vi "adc_plot.vi"(0 "Ch0":dbl[](array[numeric]), 1 "CH1":dbl[](array[numeric]), 2 "CH2":dbl[](array[numeric]), 3 "CH3":dbl[](array[numeric]), 4 "time":dbl[](array[numeric])) -> (7 "XY Graph":cluster{"time 2":dbl[], "Ch0":dbl[]}[](graph))   [LabVIEW 2022 SP3]
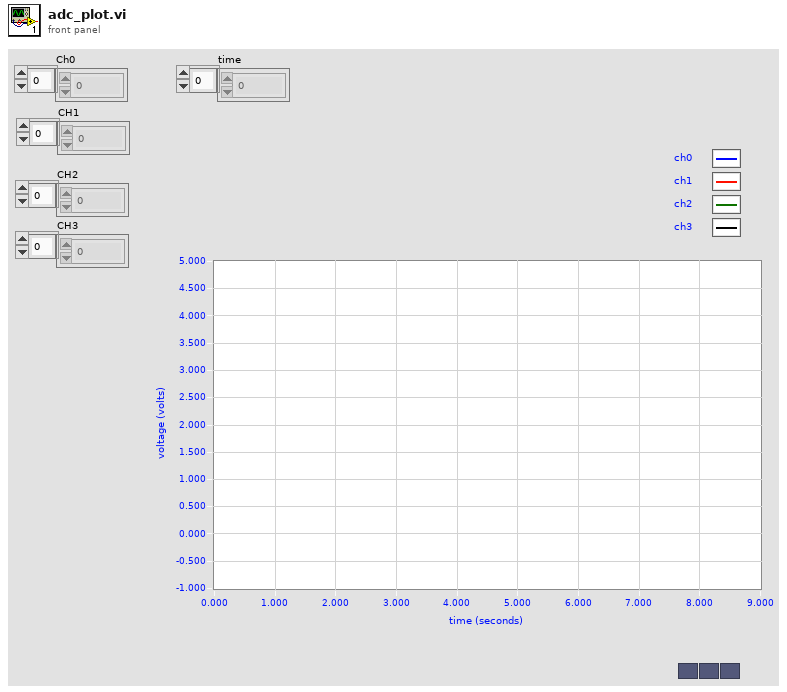
[diagram p1: front panel]
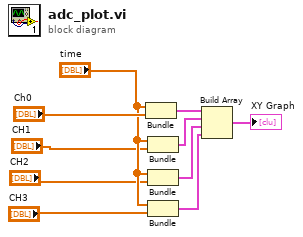
[diagram p0: block diagram]
diagram:
  n1 = Bundle("time"="time", "Ch0"="Ch0") -> (w7:cluster{"time":dbl[], "Ch0":dbl[]})  [unwired: 1 in]
  n2 = Bundle("time"="time", "CH1"="CH1") -> (w8:cluster{"time":dbl[], "CH1":dbl[]})  [unwired: 1 in]
  n3 = Bundle("time"="time", "CH2"="CH2") -> (w9:cluster{"time":dbl[], "CH2":dbl[]})  [unwired: 1 in]
  n4 = Bundle("time"="time", "CH3"="CH3") -> (w10:cluster{"time":dbl[], "CH3":dbl[]})  [unwired: 1 in]
  n5 = Build Array(w7, w8, w9, w10) -> (→"XY Graph":cluster{"time":dbl[], "CH3":dbl[]}[])
